vi "ServiceWaitState.vi"(8 "error in (no error)":errorcluster, 10 "Cluster in":T2, 11 "Enum in":T1) -> (0 "error out":errorcluster, 2 "Cluster out":T2, 3 "Enum":T1)   [LabVIEW 2018]
uses:
  Type_Def Actuator Controls.ctl
  Type_Def_Current_state_output.ctl
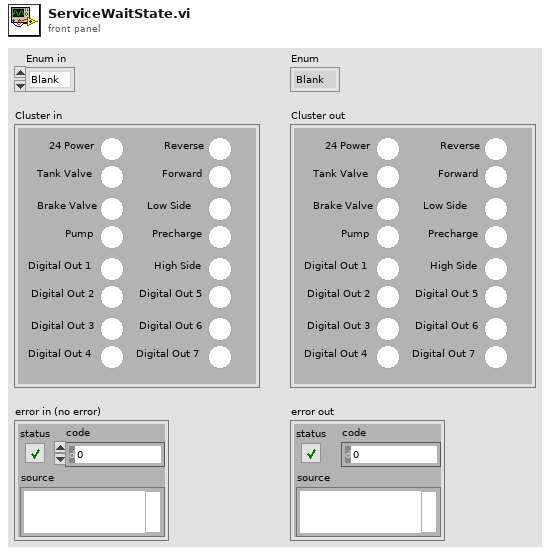
[diagram p1: front panel]
types:
  T1 = typedef "Type_Def_Current_state_output.ctl" = enum16{"Blank", "Systems Check", "Idle", "Ready", "Pushing", "CrawlingPrecharge", "Braking", "Fault", "Boot Up", "Unpowered", "Crawling", "Shutdown", "Service Push", "Service Wait", "Vent", "Precharge", "Cooldown"}
  T2 = typedef "Type_Def Actuator Controls.ctl" = cluster{"Reverse ":bool, "Forward":bool, "Low Side":bool, "Precharge":bool, "High Side":bool, "Digital Out 5":bool, "Digital Out 6":bool, "Digital Out 7 ":bool, "24 Power":bool, "Tank Valve ":bool, "Brake Valve":bool, "Pump":bool, "Digital Out 1 ":bool, "Digital Out 2":bool, "Digital Out 3":bool, "Digital Out 4 ":bool}
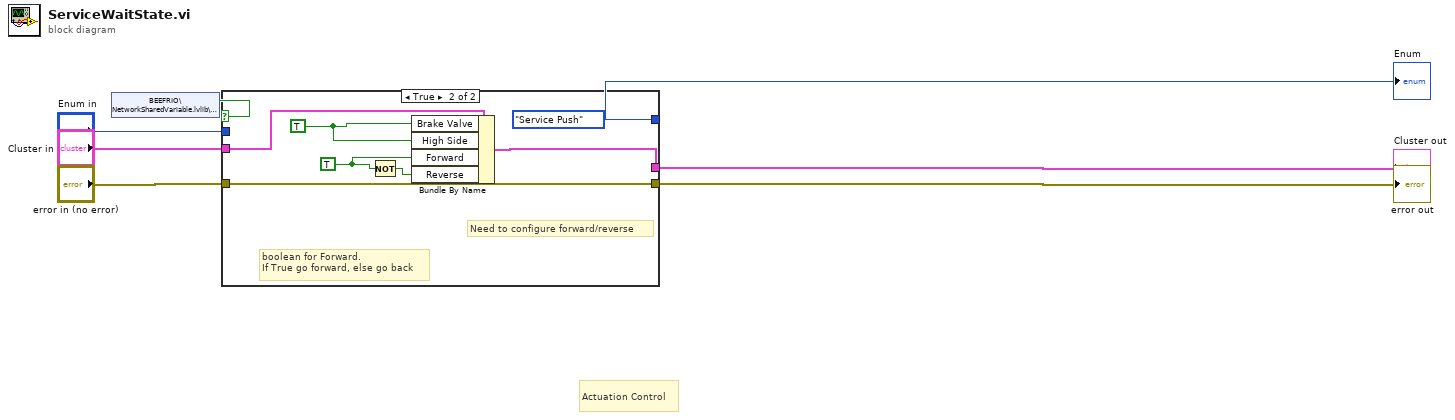
[diagram p0: block diagram]
diagram:
  # "Actuation Control"
  n1 = shared-variable "BEEFRIO\\NetworkSharedVariable.lvlib\\ServicePush"() -> (w7:bool)  [unwired: 1 in, 1 out]
  n2 = case shown="True" w7 {
    tunnel: "Enum in" -> [w10 _]
    tunnel: [w10 Type_Def_Current_state_output."Service Push"] -> w2
    tunnel: "Cluster in" -> [w9 w14]
    tunnel: [w9 w15] -> w4
    tunnel: [w8 w16] -> w5
    tunnel: "error in (no error)" -> [w8 w16]
    frame False {
    }
    frame True {
      w11 = TRUE
      w13 = TRUE ("Digital Out 5")
      # "boolean for Forward. \nIf True go forward, else go back"
      # "Need to configure forward/reverse"
      n3 = Not(x=w11) -> (.not. x?=w12:bool)
      n4 = Bundle By Name(cluster=w14, "Brake Valve"=w13, "High Side"=w13, "Forward"=w11, "Reverse"=w12) -> (w15:T2)
    }
  }
  "error out" <- w5
  "Cluster out" <- w4
  "Enum" <- w2
